vi "sub_CloseDevices.vi"(8 "error in (no error)":errorcluster, 10 "Dynamic data 2":T1, 11 "Input parameters":T2={"Measurement type"=enum."Test", "Sensor type"=enum."One channel", "Input file"="", "Output file"="test.txt", "Open after execution?"=FALSE, "Display channel"=0, "Voltage Delay (s)"=0.5, "Switch Delay (s)"=0.01, "VISA resource name source"="", "VISA resource name LCR"="", "Voltage Limit (V)"=1000.0, "Enable Voltage Auto Range (T:Enable)"=TRUE, "Voltage Manual Range (1.0)"=1.0, "Compliance  Level (uA)"=10.0} {"Voltage Limit (V)" format="%#_13g"; "Voltage Delay (s)" format="%#_13g"; "Switch Delay (s)" format="%#_13g"}) -> (0 "error out":errorcluster, 2 "Dynamic data":T1, 3 "Input parameters":T2={"Measurement type"=enum."Test", "Sensor type"=enum."One channel", "Input file"="", "Output file"="test.txt", "Open after execution?"=FALSE, "Display channel"=0, "Voltage Delay (s)"=0.5, "Switch Delay (s)"=0.01, "VISA resource name source"="", "VISA resource name LCR"="", "Voltage Limit (V)"=1000.0, "Enable Voltage Auto Range (T:Enable)"=TRUE, "Voltage Manual Range (1.0)"=1.0, "Compliance  Level (uA)"=10.0} {"Voltage Limit (V)" format="%#_13g"; "Voltage Delay (s)" format="%#_13g"; "Switch Delay (s)" format="%#_13g"})   [LabVIEW 2015]
uses:
  Program Files (x86)/National Instruments/LabVIEW 2016/instr.lib/Keithley 24XX/Keithley 24XX.lvlib
  Program Files (x86)/National Instruments/LabVIEW 2016/instr.lib/Agilent 428X Series/Agilent 428X Series.lvlib
  Input_parameters.ctl
  Dynamic_data.ctl
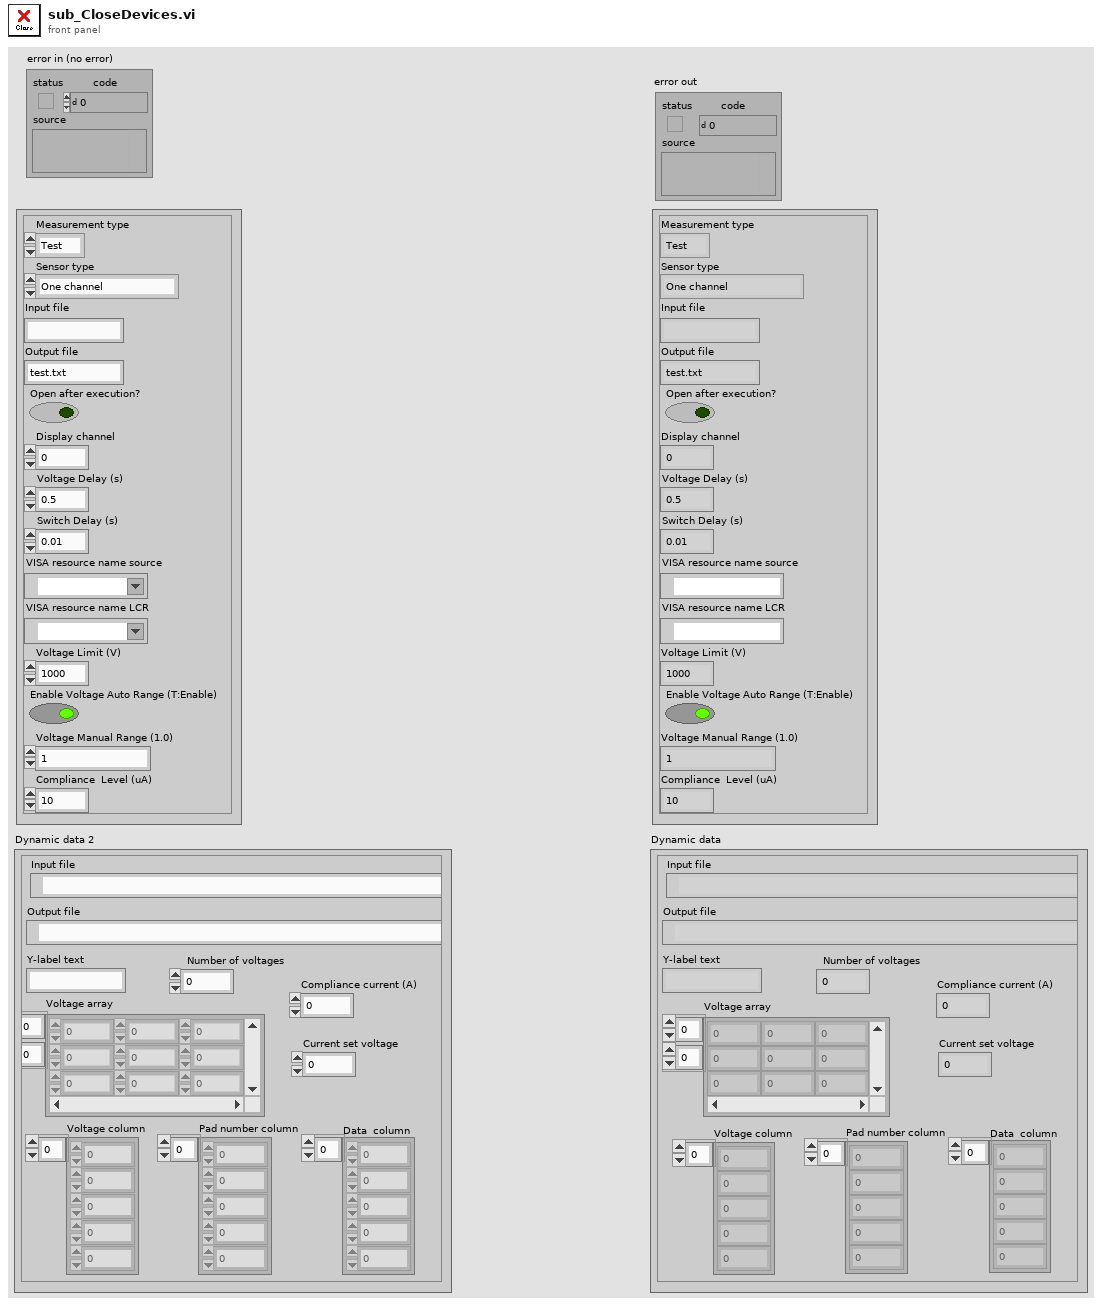
[diagram p1: front panel]
types:
  T1 = typedef "Dynamic_data.ctl" = cluster{"Input file":path, "Output file":path, "Y-label text":string, "Voltage array":dbl[][], "Current set voltage":dbl, "Voltage column":dbl[], "Pad number column":dbl[], "Data  column":dbl[], "Number of voltages":i32, "Compliance current (A)":dbl}
  T2 = typedef "Input_parameters.ctl" = cluster{"Measurement type":enum16{"IV", "CV", "Test"}, "Sensor type":enum16{"6''", "8''", "One channel"}, "Input file":string, "Output file":string, "Open after execution?":bool, "Display channel":i32, "Voltage Delay (s)":dbl, "Switch Delay (s)":dbl, "VISA resource name source":refnum<visa-resource-name>, "VISA resource name LCR":refnum<visa-resource-name>, "Voltage Limit (V)":dbl, "Enable Voltage Auto Range (T:Enable)":bool, "Voltage Manual Range (1.0)":dbl, "Compliance  Level (uA)":dbl}
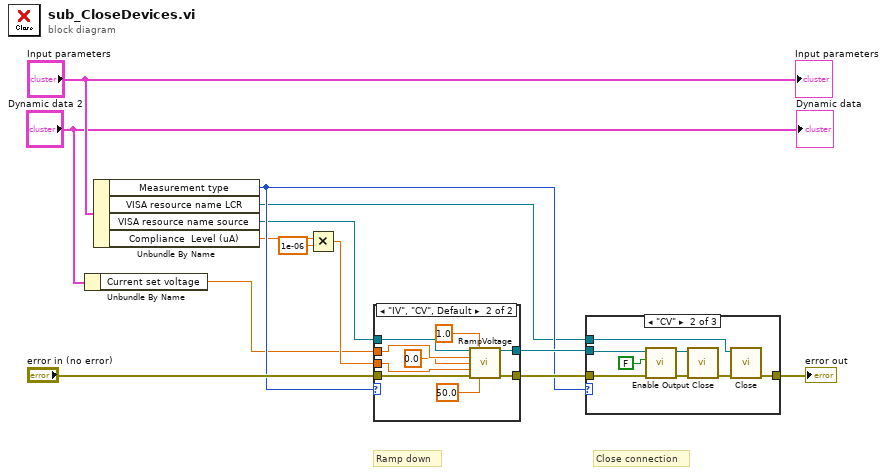
[diagram p0: block diagram]
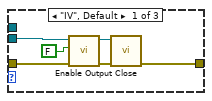
[diagram p3: hidden frame]
diagram:
  # "Close connection"
  # "Ramp down"
  n1 = Unbundle By Name("Dynamic data 2") -> ("Current set voltage"=w1:dbl)
  n2 = Unbundle By Name("Input parameters") -> ("Measurement type"=w8:enum16{"IV", "CV", "Test"}, "VISA resource name LCR"=w7:refnum<visa-resource-name>, "VISA resource name source"=w6:refnum<visa-resource-name>, "Compliance  Level (uA)"=w4:dbl)
  n3 = Multiply(x=w4, y=1e-06) -> (x*y=w3:dbl)
  n4 = case shown="\"IV\", \"CV\", Default" w8 {
    tunnel: w6 -> [w15 w21]
    tunnel: [w15 w23] -> w12
    tunnel: "error in (no error)" -> [w14 w22]
    tunnel: [w14 w24] -> w13
    tunnel: w3 -> [_ w19]
    tunnel: w1 -> [_ w20]
    frame "Test" {
    }
    frame "IV", "CV", Default {
      n5 = call "RampVoltage.vi"("VISA resource name"=w21, "Delay (s)"=1.0, "Current voltage (V)"=w20, "Target voltage (V)"=0.0, "Compliance Current (A)"=w19, "error in (no error)"=w22, "Step size (V)"=50.0) -> ("VISA resource name out"=w23:refnum<visa-resource-name>, "error out"=w24:errorcluster)  [unwired: 6 in, 1 out]
    }
  }
  n6 = case shown="\"CV\"" w8 {
    tunnel: w7 -> [_ w38 _]
    tunnel: w13 -> [w28 w31 w39]
    tunnel: [w30 w37 w39] -> w10
    tunnel: w12 -> [w27 w32 _]
    frame "IV", Default {
      n7 = call "Enable Output.vi"("error in (no error)"=w28, "Enable Output (T: Enable)"=FALSE ("Enable Output"), "VISA resource name"=w27) -> ("error out"=w25:errorcluster, "VISA resource name out"=w26:refnum<visa-resource-name>)  [unwired: 7 in]
      n8 = call "Close.vi"("error in (no error)"=w25, "VISA resource name"=w26) -> ("error out"=w30:errorcluster)  [unwired: 9 in]
    }
    frame "CV" {
      n9 = call "Enable Output.vi"("error in (no error)"=w31, "Enable Output (T: Enable)"=FALSE ("Enable Output"), "VISA resource name"=w32) -> ("error out"=w33:errorcluster, "VISA resource name out"=w34:refnum<visa-resource-name>)  [unwired: 7 in]
      n10 = call "Close.vi"("error in (no error)"=w33, "VISA resource name"=w34) -> ("error out"=w36:errorcluster)  [unwired: 9 in]
      n11 = call "Close.vi"("error in (no error)"=w36, "VISA resource name"=w38) -> ("error out"=w37:errorcluster)  [unwired: 9 in]
    }
    frame "Test" {
    }
  }
  "error out" <- w10
  "Input parameters" <- "Input parameters"
  "Dynamic data" <- "Dynamic data 2"
